vi "TAT_Com_PLC.vi"() -> ()   [LabVIEW 2017]
uses:
  Controls/PLC_Comm_State.ctl
  <vilib>/NI/Modbus Library/API/Master/Modbus Master.lvclass
  <vilib>/NI/Modbus Library/API/Wrapper/Create TCP Master.vi
  Global/PLC_to_Auto.vi
  <vilib>/NI/Modbus Library/API/Wrapper/API Main.lvlib
panel:
  in  "milliseconds to wait":u32=500
  out "error IO":errorcluster
  out "MANUAL SW":bool[](array[boolean])
  out "i/o sCREEN":bool[](array[boolean])
  out "error out 2":errorcluster
  in  "stop 2":bool
  out "Scanned Value D6000":string
  out "Write to PLC":bool[](array[boolean])
  out "error out":errorcluster
  out "Read set 1":u16[](array[numeric])
  out "PLC STATUS station 1":bool
  in  "error in":errorcluster
  in  "stop":bool
  # "STATION 1"
  # "SCAN OK\nSCAN NG \nSoftware on Bit\nRQST FRM TCO REST SCN DT"
  # "8192- 16\n8222 -10"
  # "CYCLE TIME\nAMBIENT TEMP\nBLINKER CURRENT OK\nTEMP SENSOR OK\nPART OK COUNT\nPART NOK COUNT\nFAULT BIT\nVARIENT\nHOUR\nMINUTE\nSECOND\nDAY\nMONTH\nYEAR\nSERIAL NUMBER\nShift\nAVM\nTS\nIV3"
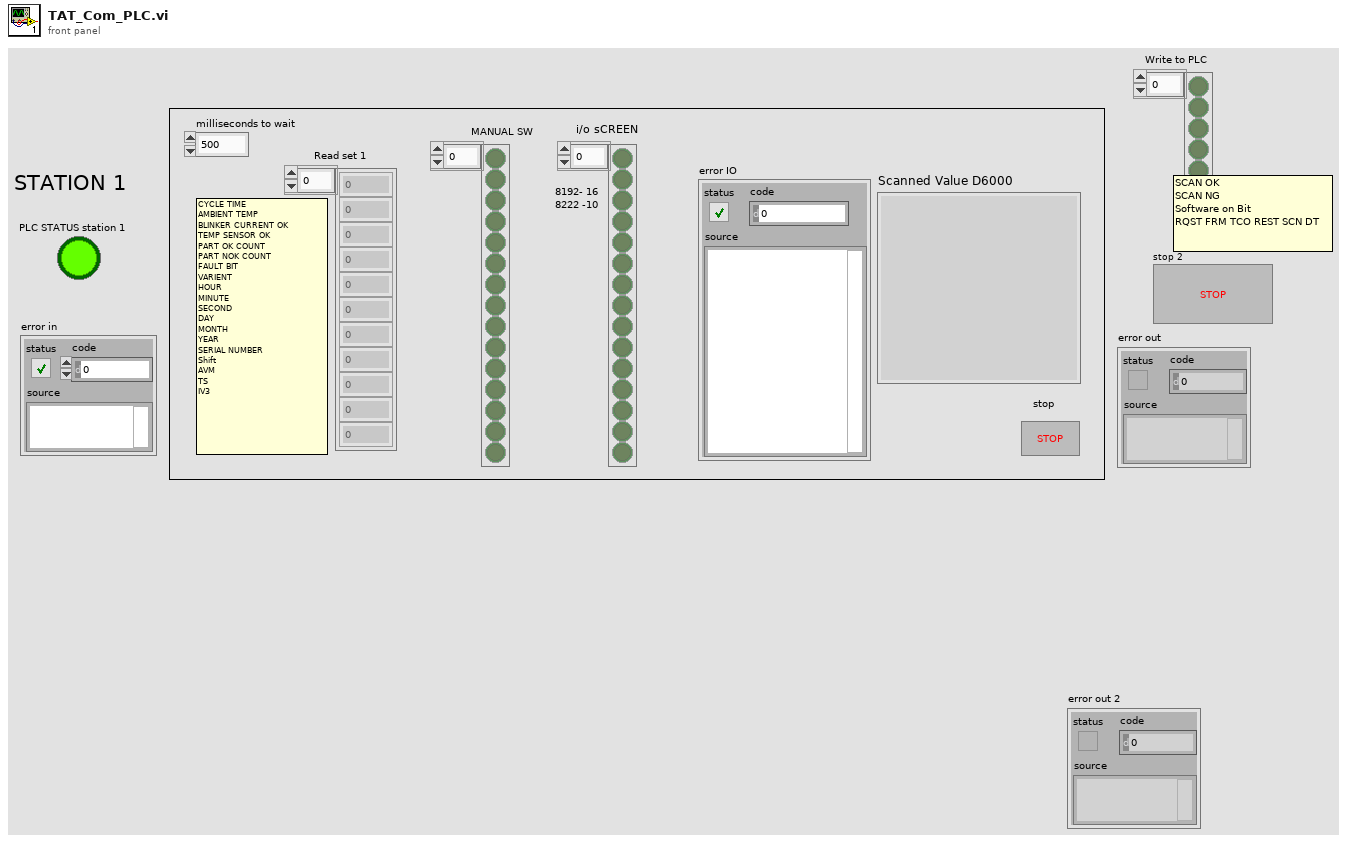
[diagram p1: front panel]
types:
  T1 = typedef "PLC_Comm_State.ctl" = enum16{"Int", "Connect", "Write", "Write2", "Write3", "Read", "Read2", "Read3", "Error", "Disconnect"}
  T2 = cluster{"RH Scanner Com Port":refnum<visa-resource-name>, "IP Address":string, "LH Scanner Com Port":refnum<visa-resource-name>}
  T3 = enum32{"invalid app kind", "Development System", "Run Time System", "Student Edition", "Embedded LabVIEW", "Evaluation", "Custom"}
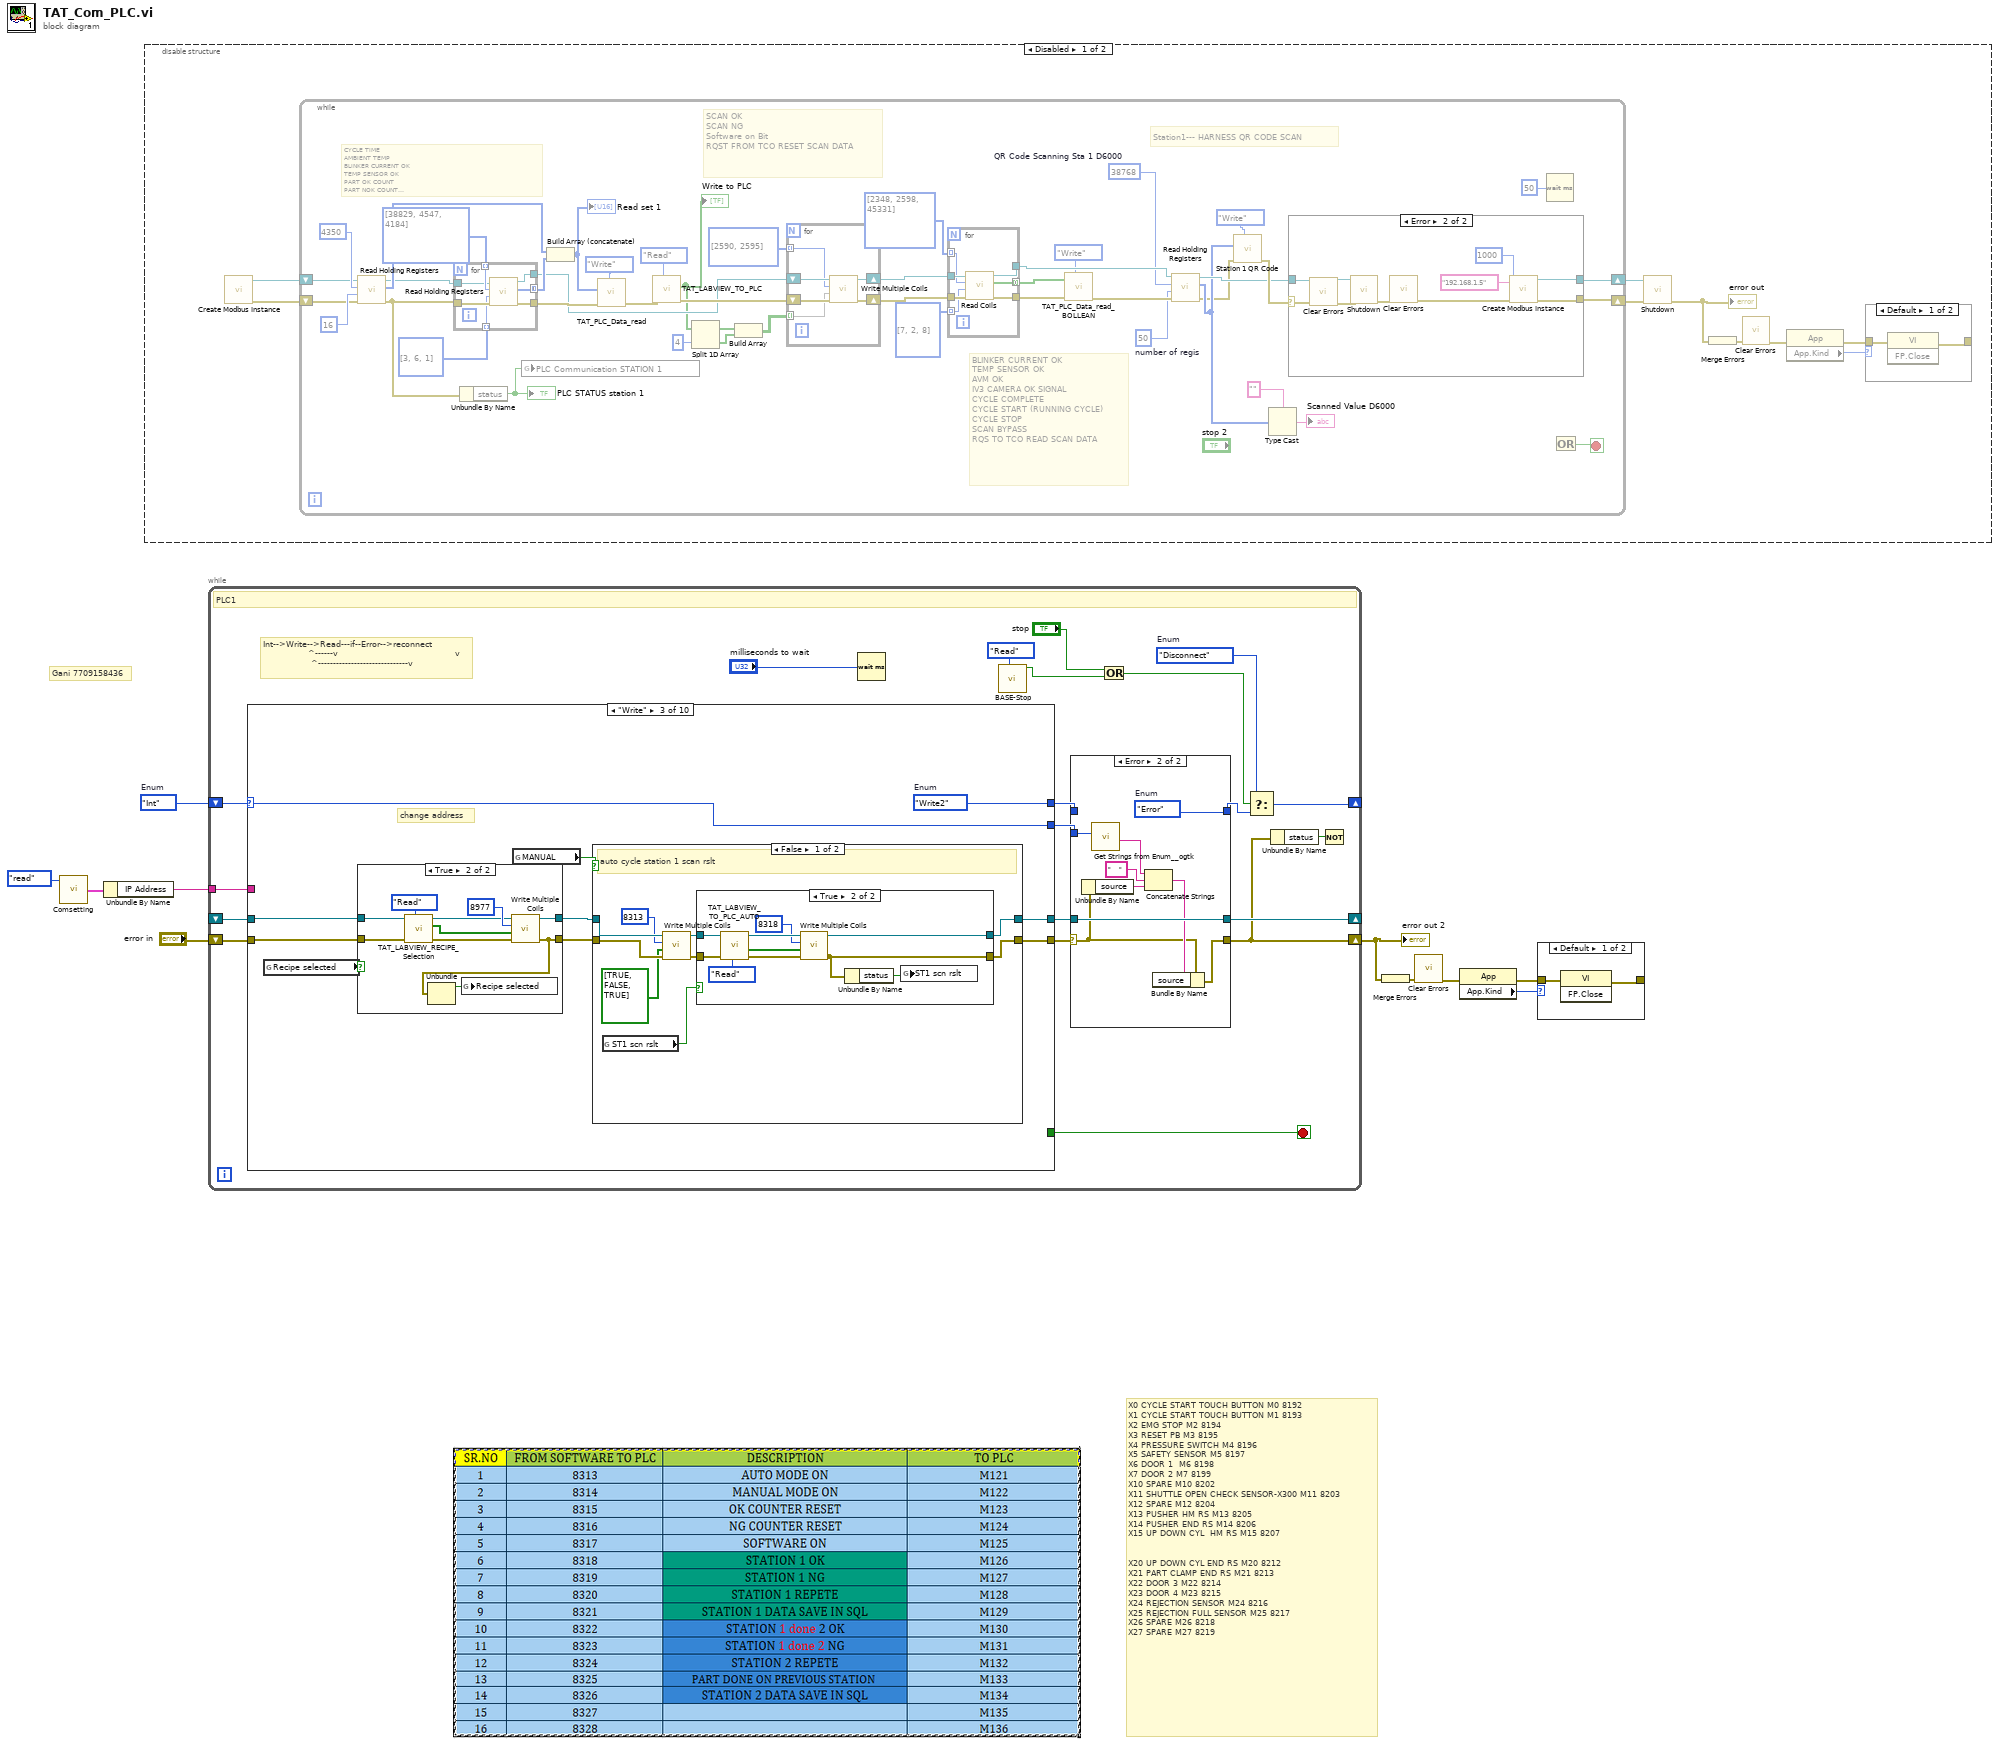
[diagram p0: block diagram]
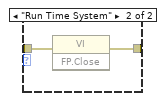
[diagram p3: hidden frame]
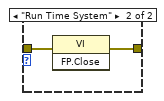
[diagram p5: hidden frame]
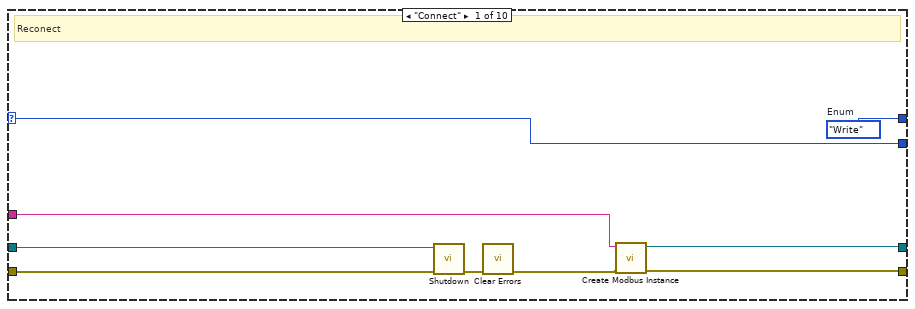
[diagram p7: hidden frame]
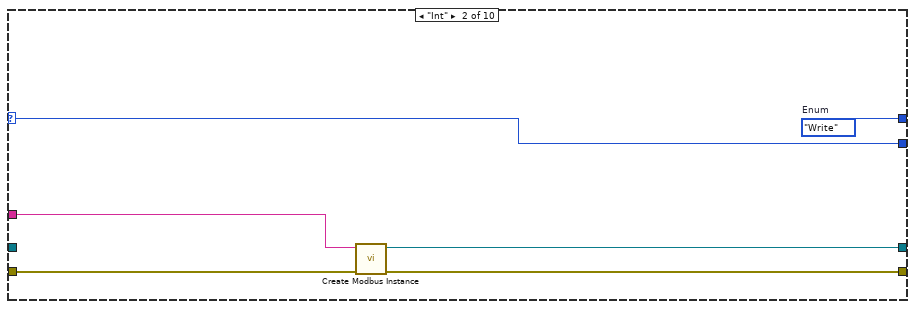
[diagram p8: hidden frame]
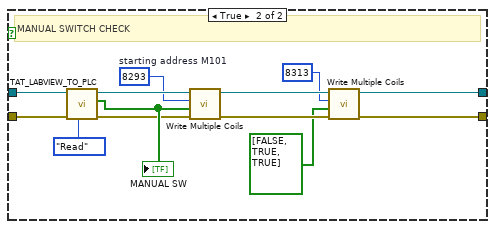
[diagram p11: hidden frame]
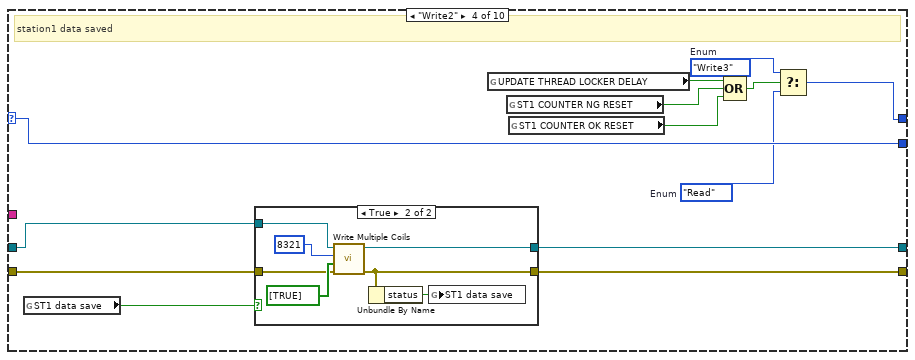
[diagram p12: hidden frame]
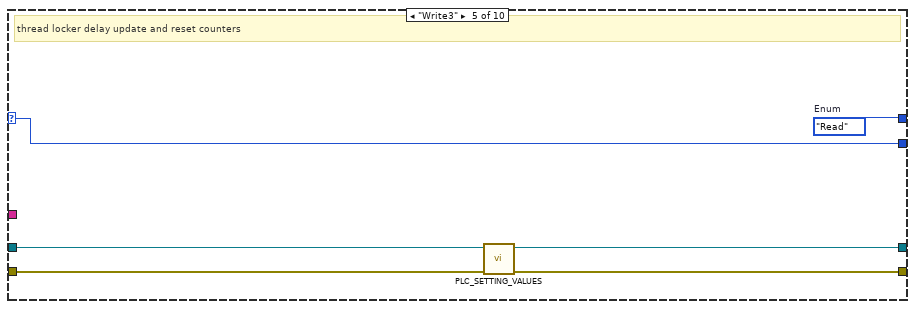
[diagram p14: hidden frame]
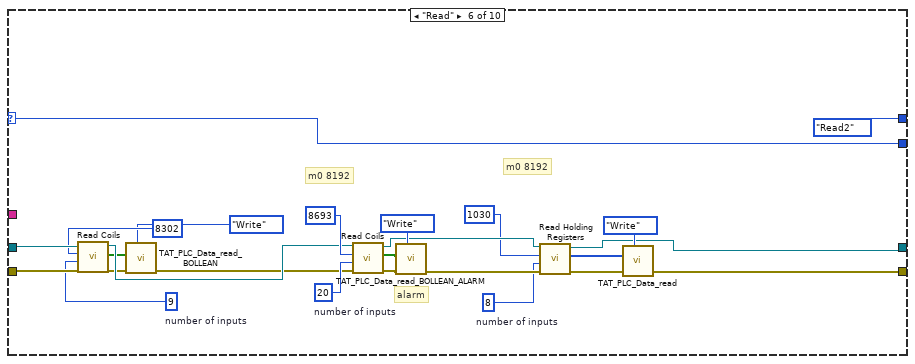
[diagram p15: hidden frame]
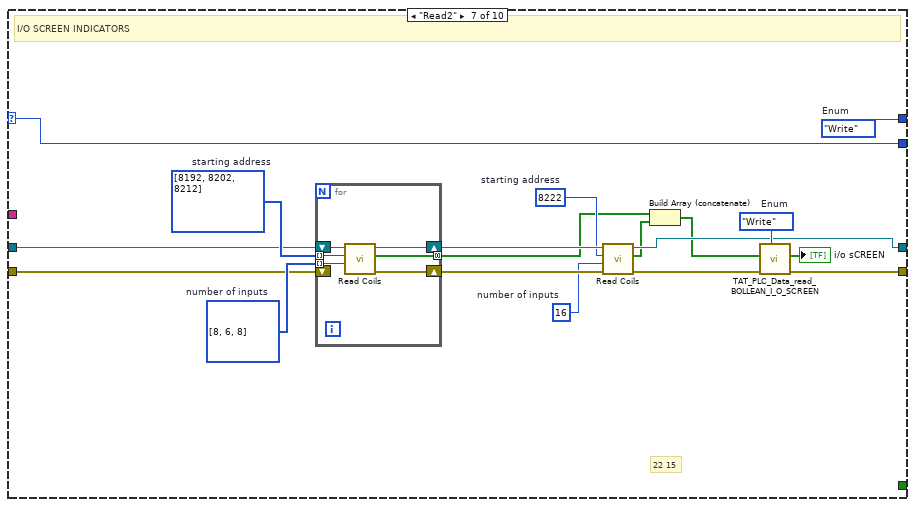
[diagram p16: hidden frame]
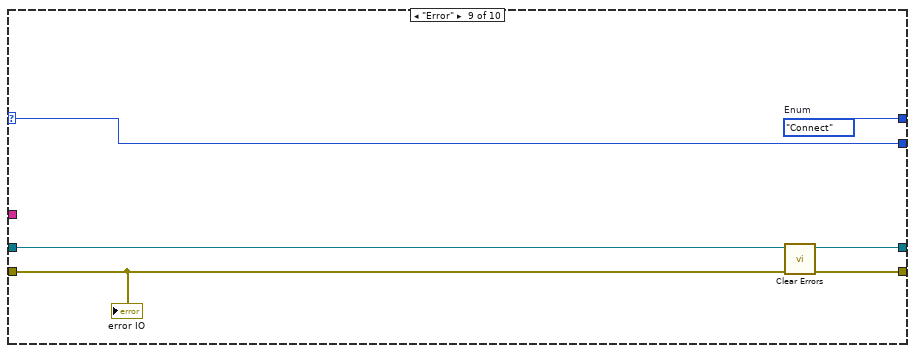
[diagram p18: hidden frame]
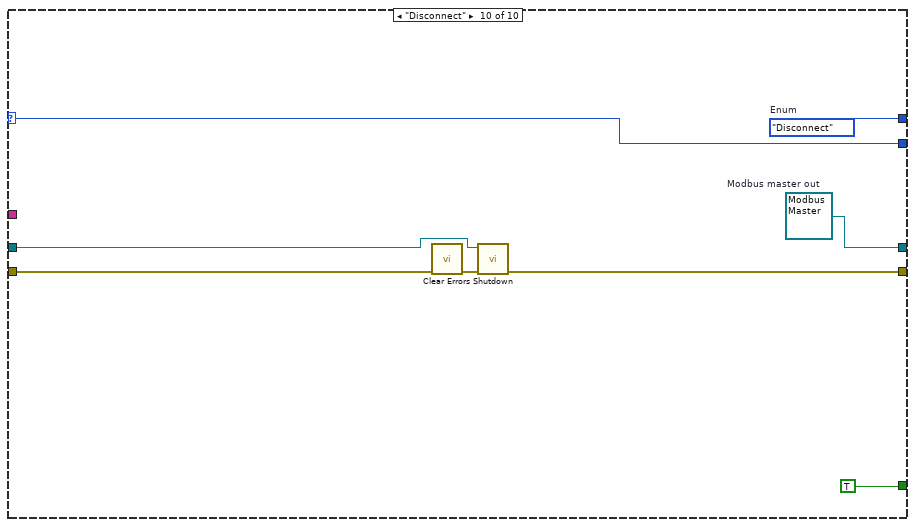
[diagram p19: hidden frame]
diagram:
  w10 = PLC_Comm_State."Int"  # Enum
  # "Gani 7709158436"
  # "X0\tCYCLE START TOUCH BUTTON\tM0\t8192\nX1\tCYCLE START TOUCH BUTTON\tM1\t8193\nX2\tEMG STOP\tM2\t8194\nX3\tRESET PB\tM3\t8195\nX4\tPRESSURE SWITCH\tM4\t8196\nX5\tSAFETY SENSOR\tM5\t8197\nX6\tDOOR 1 \tM6\t8198\nX7\tDOOR 2\tM7\t8199\nX10\tSPARE\tM10\t8202\nX11\tSHUTTLE OPEN CHECK SENSOR-X300\tM11\t8203\nX12\tSPARE\tM12\t8204\nX13\tPUSHER HM RS\tM13\t8205\nX14\tPUSHER END RS\tM14\t8206\nX15\tUP DOWN CYL  HM RS\tM15\t8207\n\t\t\t\n\t\t\t\nX20\tUP DOWN CYL END RS\tM20\t8212\nX21\tPART CLAMP END RS\tM21\t8213\nX22\tDOOR 3\tM22\t8214\nX23\tDOOR 4\tM23\t8215\nX24\tREJECTION SENSOR\tM24\t8216\nX25\tREJECTION FULL SENSOR\tM25\t8217\nX26\tSPARE\tM26\t8218\nX27\tSPARE\tM27\t8219"
  n1 = call "Comsetting.vi"("Enum"=enum16{"read", "write"}."read") -> ("Cluster Out"=w2:T2)  [unwired: 2 in, 2 out]
  n2 = Unbundle By Name(w2) -> ("IP Address"=w1:string)
  n3 = disable-structure shown="Disabled" {
    frame Disabled {
      n4 = call-poly <vilib>:"Create Modbus Instance.vi"() -> ("error out"=w15:errorcluster, "TCP master instance"=w14:refnum<class "Modbus Master.lvclass">)  [unwired: 10 in]
      n5 = while {
        shift-right: [w64] -> w19
        shift-left: w14 -> [w26]
        shift-right: [w63] -> w18
        shift-left: w15 -> [w27]
        stop <- w65 stop-if-true
        w46 = u16 50  # number of regis
        w47 = u16 38768  # QR Code Scanning Sta 1 D6000
        # "SCAN OK\nSCAN NG \nSoftware on Bit\nRQST FROM TCO RESET SCAN DATA"
        # "BLINKER CURRENT OK\nTEMP SENSOR OK\nAVM OK\nIV3 CAMERA OK SIGNAL\nCYCLE COMPLETE\nCYCLE START (RUNNING CYCLE)\nCYCLE STOP\nSCAN BYPASS\nRQS TO TCO READ SCAN DATA"
        # "Station1--- HARNESS QR CODE SCAN"
        # "CYCLE TIME\nAMBIENT TEMP\nBLINKER CURRENT OK\nTEMP SENSOR OK\nPART OK COUNT\nPART NOK COUNT\nFAULT BIT\nVARIENT\nHOUR\nMINUTE\nSECOND\nDAY\nMONTH\nYEAR\nSERIAL NUMBER\nShift\nAVM\nTS\nIV3 CAMERA"
        n6 = call-dynamic "Read Holding Registers.vi"("error in"=w27, "number of inputs"=u16 16, "starting address"=u16 4350 ("starting address 2"), "Modbus master in"=w26) -> ("error out"=w38:errorcluster, "register values"=w32:u16[], "Modbus master out"=w30:refnum<class "Modbus Master.lvclass">)  [unwired: 5 in]
        n7 = for {
          tunnel: u16[] [38829, 4547, 4184] ("starting address 2") -> [w95] mode=indexing
          tunnel: u16[] [3, 6, 1] ("number of inputs") -> [w94] mode=indexing
          tunnel: [w92] -> w31 mode=concatenating
          tunnel: w30 -> [w91]
          tunnel: [w90] -> w29
          tunnel: w38 -> [w96]
          tunnel: [w93] -> w34
          n8 = call-dynamic "Read Holding Registers.vi"("error in"=w96, "number of inputs"=w94, "starting address"=w95, "Modbus master in"=w91) -> ("error out"=w93:errorcluster, "register values"=w92:u16[], "Modbus master out"=w90:refnum<class "Modbus Master.lvclass">)  [unwired: 5 in]
        }
        n9 = Unbundle By Name(w38) -> ("status"=w55:bool)
        "PLC STATUS station 1" <- w55
        n10 = global write "PLC_to_Auto.vi" "PLC Communication STATION 1"(w55) -> ()
        n11 = Build Array (concatenate)(w32, w31) -> (w28:u16[])
        "Read set 1" <- w28
        n12 = call "TAT_PLC_Data_read.vi"("Enum"=enum16{"Read", "Write"}."Write", "error in (no error)"=w34, "Array"=w28) -> ("error out"=w33:errorcluster)  [unwired: 7 in, 1 out]
        n13 = call "TAT_LABVIEW_TO_PLC.vi"("Enum"=enum16{"Read", "Write"}."Read", "error in (no error)"=w33) -> ("error out"=w58:errorcluster, "Array 2"=w24:bool[])  [unwired: 8 in]
        "Write to PLC" <- w24
        n14 = Split 1D Array(array=w24, index=4) -> (first subarray=w23:bool[], second subarray=w22:bool[])
        n15 = Build Array(w23, w22) -> (w21:bool[][])
        n16 = for {
          tunnel: w21 -> [w88] mode=indexing
          shift-right: [w87] -> w57
          shift-left: w58 -> [w89]
          shift-right: [w86] -> w56
          shift-left: w29 -> [w85]
          tunnel: u16[] [2590, 2595] ("starting address") -> [w84] mode=indexing
          n17 = call-dynamic "Write Multiple Coils.vi"("error in"=w89, "coils to write"=w88, "starting address"=w84, "Modbus master in"=w85) -> ("error out"=w87:errorcluster, "Modbus master out"=w86:refnum<class "Modbus Master.lvclass">)  [unwired: 6 in]
        }
        n18 = for {
          tunnel: u16[] [7, 2, 8] ("number of inputs 2") -> [w69] mode=indexing
          tunnel: u16[] [2348, 2598, 45331] ("starting address 3") -> [w68] mode=indexing
          tunnel: w57 -> [w72]
          tunnel: [w67] -> w42
          tunnel: w56 -> [w71]
          tunnel: [w70] -> w49
          tunnel: [w66] -> w41 mode=concatenating
          n19 = call-dynamic "Read Coils.vi"("error in"=w72, "number of inputs"=w69, "starting address"=w68, "Modbus master in"=w71) -> ("error out"=w67:errorcluster, "coils"=w66:bool[], "Modbus master out"=w70:refnum<class "Modbus Master.lvclass">)  [unwired: 5 in]
        }
        n20 = call "TAT_PLC_Data_read_BOLLEAN.vi"("Enum"=enum16{"Read", "Write"}."Write", "error in (no error)"=w42, "Array"=w41) -> ("error out"=w50:errorcluster)  [unwired: 7 in, 1 out]
        n21 = call-dynamic "Read Holding Registers.vi"("error in"=w50, "number of inputs"=w46, "starting address"=w47, "Modbus master in"=w49) -> ("error out"=w39:errorcluster, "register values"=w40:u16[], "Modbus master out"=w48:refnum<class "Modbus Master.lvclass">)  [unwired: 5 in]
        n22 = call "Station 1 QR Code.vi"("Enum"=enum16{"Read", "Write"}."Write", "error in (no error)"=w39, "Array"=w40) -> ("error out"=w51:errorcluster)  [unwired: 7 in, 1 out]
        n23 = Type Cast(type="", x=w40) -> (*(type *) &x=→"Scanned Value D6000":string)
        n24 = case shown="Error" w51 {
          selector: w51 -> [w73 w83]
          tunnel: w48 -> [w74 w81]
          tunnel: [w74 w77] -> w64
          tunnel: [w73 w76] -> w63
          frame No Error {
          }
          frame Error {
            n25 = call <vilib>:"Clear Errors.vi"("error in (no error)"=w83) -> ("error out"=w82:errorcluster)  [unwired: 5 in, 1 out]
            n26 = call-dynamic "Shutdown.vi"("error in"=w82, "Modbus master in"=w81) -> ("error out"=w80:errorcluster)  [unwired: 9 in]
            n27 = call <vilib>:"Clear Errors.vi"("error in (no error)"=w80) -> ("error out"=w78:errorcluster)  [unwired: 5 in, 1 out]
            n28 = call-poly <vilib>:"Create Modbus Instance.vi"("error in"=w78, "connect timeout ms"=1000, "address"="192.168.1.5") -> ("error out"=w76:errorcluster, "TCP master instance"=w77:refnum<class "Modbus Master.lvclass">)  [unwired: 7 in]
          }
        }
        n29 = Wait (ms)(milliseconds to wait=u32 50) -> ()  [unwired: 1 out]
        n30 = Or() -> (x .or. y?=w65:bool)  [unwired: 2 in]
      }
      n31 = call-dynamic "Shutdown.vi"("error in"=w18, "Modbus master in"=w19) -> ("error out"=w12:errorcluster)  [unwired: 9 in]
      "error out" <- w12
      n32 = Merge Errors(w12) -> (w11:errorcluster)
      n33 = call <vilib>:"Clear Errors.vi"("error in (no error)"=w11) -> ("error out"=w13:errorcluster)  [unwired: 5 in, 1 out]
      n34 = property class="App"(error in=w13) -> (error out=w16:errorcluster, "App.Kind"=w17:T3)  [unwired: 1 in, 1 out]
      n35 = case shown="Default" w17 {
        tunnel: w16 -> [w98 w100]
        tunnel: [w97 w99] -> _
        frame Default {
          n36 = invoke class="VI" method="FP.Close"(error in=w98) -> (error out=w97:errorcluster)  [unwired: 2 in, 2 out]
        }
        frame "Run Time System" {
          n37 = invoke class="VI" method="FP.Close"(error in=w100) -> (error out=w99:errorcluster)  [unwired: 2 in, 2 out]
        }
      }
    }
    frame Enabled {
    }
  }
  n38 = while {
    shift-right: [w110] -> _
    shift-left: w10 -> [w119]
    shift-right: [w105] -> w4
    shift-left: "error in" -> [w118]
    shift-right: [w113] -> _
    shift-left: _ -> [w117]
    tunnel: w1 -> [w116]
    stop <- w111 stop-if-true
    w101 = PLC_Comm_State."Disconnect"  # Enum
    # "Int-->Write-->Read---if--Error-->reconnect\n               ^------v                                       v\n                ^------------------------------v"
    # "PLC1"
    n39 = case shown="\"Write\"" w119 {
      selector: w119 -> [w141 w146 w157 w213 w227 w252 w261 _ w281 w289]
      tunnel: [w138 w142 w156 w208 w223 w234 w264 w278 w282 w286] -> w120
      tunnel: [w136 w143 w155 w209 w225 w232 w259 w277 w283 w284] -> w112
      tunnel: w118 -> [w135 w147 w151 w210 w224 w250 w257 w278 w279 w291]
      tunnel: w117 -> [w133 _ w149 w211 w226 w251 w260 w277 w283 w285]
      tunnel: w116 -> [w137 w144 _ _ _ _ _ _ _ _]
      tunnel: [w140 w145 w153 w207 w228 PLC_Comm_State."Read2" ("Enum") w262 _ w280 w288] -> w114
      tunnel: [_ _ _ _ _ _ _ _ _ TRUE] -> w111
      tunnel: [w141 w146 w157 w213 w227 w252 w261 _ w281 w289] -> w108
      frame "Connect" {
        w140 = PLC_Comm_State."Write"  # Enum
        # "Reconect"
        n40 = call-dynamic "Shutdown.vi"("error in"=w135, "Modbus master in"=w133) -> ("error out"=w134:errorcluster)  [unwired: 9 in]
        n41 = call <vilib>:"Clear Errors.vi"("error in (no error)"=w134) -> ("error out"=w139:errorcluster)  [unwired: 5 in, 1 out]
        n42 = call-poly <vilib>:"Create Modbus Instance.vi"("error in"=w139, "address"=w137) -> ("error out"=w138:errorcluster, "TCP master instance"=w136:refnum<class "Modbus Master.lvclass">)  [unwired: 8 in]
      }
      frame "Int" {
        w145 = PLC_Comm_State."Write"  # Enum
        n43 = call-poly <vilib>:"Create Modbus Instance.vi"("error in"=w147, "address"=w144) -> ("error out"=w142:errorcluster, "TCP master instance"=w143:refnum<class "Modbus Master.lvclass">)  [unwired: 8 in]
      }
      frame "Write" {
        w153 = PLC_Comm_State."Write2"  # Enum
        # "change address"
        n44 = global read "PLC_to_Auto.vi" "Recipe selected"() -> (w148:bool)
        n45 = case shown="True" w148 {
          tunnel: [w158 w165] -> w152
          tunnel: w151 -> [w158 w162]
          tunnel: [w159 w167] -> w150
          tunnel: w149 -> [w159 w166]
          frame False {
          }
          frame True {
            n46 = call "TAT_LABVIEW_RECIPE_Selection.vi"("Enum"=enum16{"Read", "Write"}."Read", "error in (no error)"=w162) -> ("error out"=w163:errorcluster, "Array 2"=w160:bool[])  [unwired: 8 in]
            n47 = call-dynamic "Write Multiple Coils.vi"("error in"=w163, "coils to write"=w160, "starting address"=u16 8977, "Modbus master in"=w166) -> ("error out"=w165:errorcluster, "Modbus master out"=w167:refnum<class "Modbus Master.lvclass">)  [unwired: 6 in]
            n48 = Unbundle(w165) -> ("status"=w164:bool)  [unwired: 2 out]
            n49 = global write "PLC_to_Auto.vi" "Recipe selected"(w164) -> ()
          }
        }
        n50 = global read "PLC_to_Auto.vi" "MANUAL"() -> (w154:bool)
        n51 = case shown="False" w154 {
          tunnel: w152 -> [w177 w196]
          tunnel: [w169 w191] -> w156
          tunnel: w150 -> [w176 w200]
          tunnel: [w170 w193] -> w155
          frame False {
            # "auto cycle station 1 scan rslt"
            n52 = global read "PLC_to_Auto.vi" "ST1 scn rslt"() -> (w173:bool)
            n53 = call-dynamic "Write Multiple Coils.vi"("error in"=w177, "coils to write"=bool[] [TRUE, FALSE, TRUE], "starting address"=u16 8313 ("starting address M101"), "Modbus master in"=w176) -> ("error out"=w172:errorcluster, "Modbus master out"=w171:refnum<class "Modbus Master.lvclass">)  [unwired: 6 in]
            n54 = case shown="True" w173 {
              tunnel: w172 -> [w179 w188]
              tunnel: w171 -> [w178 w187]
              tunnel: [w178 w186] -> w170
              tunnel: [w179 w180] -> w169
              frame False {
              }
              frame True {
                n55 = call "TAT_LABVIEW_TO_PLC_AUTO.vi"("Enum"=enum16{"Read", "Write"}."Read", "error in (no error)"=w188) -> ("error out"=w184:errorcluster, "Array 2"=w182:bool[])  [unwired: 8 in]
                n56 = call-dynamic "Write Multiple Coils.vi"("error in"=w184, "coils to write"=w182, "starting address"=u16 8318, "Modbus master in"=w187) -> ("error out"=w180:errorcluster, "Modbus master out"=w186:refnum<class "Modbus Master.lvclass">)  [unwired: 6 in]
                n57 = Unbundle By Name(w180) -> ("status"=w181:bool)
                n58 = global write "PLC_to_Auto.vi" "ST1 scn rslt"(w181) -> ()
              }
            }
          }
          frame True {
            w199 = u16 8293  # starting address M101
            # "MANUAL SWITCH CHECK"
            n59 = call "TAT_LABVIEW_TO_PLC.vi"("Enum"=enum16{"Read", "Write"}."Read", "error in (no error)"=w196) -> ("error out"=w195:errorcluster, "Array 2"=w197:bool[])  [unwired: 8 in]
            "MANUAL SW" <- w197
            n60 = call-dynamic "Write Multiple Coils.vi"("error in"=w195, "coils to write"=w197, "starting address"=w199, "Modbus master in"=w200) -> ("error out"=w192:errorcluster, "Modbus master out"=w194:refnum<class "Modbus Master.lvclass">)  [unwired: 6 in]
            n61 = call-dynamic "Write Multiple Coils.vi"("error in"=w192, "coils to write"=bool[] [FALSE, TRUE, TRUE], "starting address"=u16 8313 ("starting address M101"), "Modbus master in"=w194) -> ("error out"=w191:errorcluster, "Modbus master out"=w193:refnum<class "Modbus Master.lvclass">)  [unwired: 6 in]
          }
        }
      }
      frame "Write2" {
        w205 = PLC_Comm_State."Read"  # Enum
        w206 = PLC_Comm_State."Write3"  # Enum
        # "station1 data saved"
        n62 = global read "PLC_to_Auto.vi" "ST1 data save"() -> (w212:bool)
        n63 = case shown="True" w212 {
          tunnel: [w215 w222] -> w209
          tunnel: [w214 w217] -> w208
          tunnel: w211 -> [w215 w219]
          tunnel: w210 -> [w214 w218]
          frame False {
          }
          frame True {
            n64 = call-dynamic "Write Multiple Coils.vi"("error in"=w218, "coils to write"=bool[] [TRUE], "starting address"=u16 8321, "Modbus master in"=w219) -> ("error out"=w217:errorcluster, "Modbus master out"=w222:refnum<class "Modbus Master.lvclass">)  [unwired: 6 in]
            n65 = Unbundle By Name(w217) -> ("status"=w216:bool)
            n66 = global write "PLC_to_Auto.vi" "ST1 data save"(w216) -> ()
          }
        }
        n67 = global read "PLC_to_Auto.vi" "UPDATE THREAD LOCKER DELAY"() -> (w204:bool)
        n68 = global read "PLC_to_Auto.vi" "ST1 COUNTER NG RESET"() -> (w203:bool)
        n69 = global read "PLC_to_Auto.vi" "ST1 COUNTER OK RESET"() -> (w202:bool)
        n70 = Compound Arithmetic op=OR(w204, w203, w202) -> (w201:bool)
        n71 = Select(t=w206, s=w201, f=w205) -> (s? t:f=w207:T1)
      }
      frame "Write3" {
        w228 = PLC_Comm_State."Read"  # Enum
        # "thread locker delay update and reset counters"
        n72 = call "PLC_SETTING_VALUES.vi"("error in (no error)"=w224, "Modbus Master in"=w226) -> ("error out"=w223:errorcluster, "Modbus Master out"=w225:refnum<class "Modbus Master.lvclass">)  [unwired: 8 in]
      }
      frame "Read" {
        w231 = u16 8  # number of inputs
        w244 = u16 9  # number of inputs
        w248 = u16 20  # number of inputs
        # "m0 8192"
        # "m0 8192"
        # "alarm"
        n73 = call-dynamic "Read Coils.vi"("error in"=w250, "number of inputs"=w244, "starting address"=u16 8302, "Modbus master in"=w251) -> ("error out"=w241:errorcluster, "coils"=w238:bool[], "Modbus master out"=w242:refnum<class "Modbus Master.lvclass">)  [unwired: 5 in]
        n74 = call "TAT_PLC_Data_read_BOLLEAN.vi"("Enum"=enum16{"Read", "Write"}."Write", "error in (no error)"=w241, "Array"=w238) -> ("error out"=w240:errorcluster)  [unwired: 7 in, 1 out]
        n75 = call-dynamic "Read Coils.vi"("error in"=w240, "number of inputs"=w248, "starting address"=u16 8693, "Modbus master in"=w242) -> ("error out"=w247:errorcluster, "coils"=w246:bool[], "Modbus master out"=w233:refnum<class "Modbus Master.lvclass">)  [unwired: 5 in]
        n76 = call "TAT_PLC_Data_read_BOLLEAN_ALARM.vi"("Enum"=enum16{"Read", "Write"}."Write", "error in (no error)"=w247, "Array"=w246) -> ("error out"=w235:errorcluster)  [unwired: 7 in, 1 out]
        n77 = call-dynamic "Read Holding Registers.vi"("error in"=w235, "number of inputs"=w231, "starting address"=u16 1030, "Modbus master in"=w233) -> ("error out"=w234:errorcluster, "register values"=w229:u16[], "Modbus master out"=w232:refnum<class "Modbus Master.lvclass">)  [unwired: 5 in]
        n78 = call "TAT_PLC_Data_read.vi"("Enum"=enum16{"Read", "Write"}."Write", "Array"=w229) -> ()  [unwired: 8 in, 2 out]
      }
      frame "Read2" {
        w262 = PLC_Comm_State."Write"  # Enum
        w263 = enum16{"Read", "Write"}."Write"  # Enum
        w268 = u16 16  # number of inputs
        w267 = u16 8222  # starting address
        w266 = u16[] [8, 6, 8]  # number of inputs
        w265 = u16[] [8192, 8202, 8212]  # starting address
        # "22 15"
        # "I/O SCREEN INDICATORS"
        n79 = for {
          tunnel: [w274] -> w254 mode=concatenating
          tunnel: w266 -> [w273] mode=indexing
          tunnel: w265 -> [w272] mode=indexing
          shift-right: [w276] -> w270
          shift-left: w260 -> [w271]
          shift-right: [w275] -> w269
          shift-left: w257 -> [_]
          n80 = call-dynamic "Read Coils.vi"("number of inputs"=w273, "starting address"=w272, "Modbus master in"=w271) -> ("error out"=w275:errorcluster, "coils"=w274:bool[], "Modbus master out"=w276:refnum<class "Modbus Master.lvclass">)  [unwired: 6 in]
        }
        n81 = call-dynamic "Read Coils.vi"("error in"=w269, "number of inputs"=w268, "starting address"=w267, "Modbus master in"=w270) -> ("error out"=w256:errorcluster, "coils"=w255:bool[], "Modbus master out"=w259:refnum<class "Modbus Master.lvclass">)  [unwired: 5 in]
        n82 = Build Array (concatenate)(w254, w255) -> (w253:bool[])
        n83 = call "TAT_PLC_Data_read_BOLLEAN_I_O_SCREEN.vi"("Enum"=w263, "error in (no error)"=w256, "Array"=w253) -> ("error out"=w264:errorcluster, "Array 2"=→"i/o sCREEN":bool[])  [unwired: 7 in]
      }
      frame "Read3" {
        # "No Use"
      }
      frame "Error" {
        w280 = PLC_Comm_State."Connect"  # Enum
        n84 = call <vilib>:"Clear Errors.vi"("error in (no error)"=w279) -> ("error out"=w282:errorcluster)  [unwired: 5 in, 1 out]
        "error IO" <- w279
      }
      frame "Disconnect" {
        w284 = refnum<class "Modbus Master.lvclass"> refnum  # Modbus master out
        w288 = PLC_Comm_State."Disconnect"  # Enum
        n85 = call <vilib>:"Clear Errors.vi"("error in (no error)"=w291) -> ("error out"=w287:errorcluster)  [unwired: 5 in, 1 out]
        n86 = call-dynamic "Shutdown.vi"("error in"=w287, "Modbus master in"=w285) -> ("error out"=w286:errorcluster)  [unwired: 9 in]
      }
    }
    n87 = Wait (ms)(milliseconds to wait="milliseconds to wait") -> ()  [unwired: 1 out]
    n88 = call "BASE-Stop.vi"("Enum"=enum16{"Read", "Write"}."Read") -> ("Stop"=w103:bool)  [unwired: 10 in]
    n89 = case shown="Error" w120 {
      selector: w120 -> [w123 w126]
      tunnel: [w123 w125] -> w105
      tunnel: [w122 w124] -> w109
      tunnel: w114 -> [w122 _]
      tunnel: [w121 w132] -> w113
      tunnel: w112 -> [w121 w132]
      tunnel: w108 -> [_ w130]
      frame No Error {
      }
      frame Error {
        w124 = PLC_Comm_State."Error"  # Enum
        n90 = Unbundle By Name(w126) -> ("source"=w131:string)
        n91 = call <userlib>:"Get Strings from Enum__ogtk.vi"("Enum"=w130) -> ("String Value"=w129:string)  [unwired: 7 in, 3 out]
        n92 = Concatenate Strings(w129, "    " ("string"), w131) -> (w127:string)
        n93 = Bundle By Name(cluster=w126, "source"=w127) -> (w125:errorcluster)
      }
    }
    n94 = Or(x="stop", y=w103) -> (x .or. y?=w107:bool)
    n95 = Select(t=w101, s=w107, f=w109) -> (s? t:f=w110:T1)
    n96 = Unbundle By Name(w105) -> ("status"=w106:bool)
    n97 = Not(x=w106) -> ()  [unwired: 1 out]
  }
  "error out 2" <- w4
  n98 = Merge Errors(w4) -> (w8:errorcluster)
  n99 = call <vilib>:"Clear Errors.vi"("error in (no error)"=w8) -> ("error out"=w7:errorcluster)  [unwired: 5 in, 1 out]
  n100 = property class="App"(error in=w7) -> (error out=w6:errorcluster, "App.Kind"=w5:T3)  [unwired: 1 in, 1 out]
  n101 = case shown="Default" w5 {
    tunnel: w6 -> [w293 w295]
    tunnel: [w292 w294] -> _
    frame Default {
      n102 = invoke class="VI" method="FP.Close"(error in=w293) -> (error out=w292:errorcluster)  [unwired: 2 in, 2 out]
    }
    frame "Run Time System" {
      n103 = invoke class="VI" method="FP.Close"(error in=w295) -> (error out=w294:errorcluster)  [unwired: 2 in, 2 out]
    }
  }
